vi "Aero_Tunnel_Monitor.vi"() -> ()   [LabVIEW 2012]
uses:
  ATE_Road_Data.ctl
  ATE_Machine_Status.ctl
  ATE_Road_Control.ctl
  ATE_Balance_Data.ctl
  ATE_Fan_Control.ctl
  ATE_Fan_Data.ctl
  Controls/Post_Process.ctl
  <vilib>/Platform/TimedLoop/XDataNode/timing_clust.ctl
  <vilib>/Platform/TimedLoop/XDataNode/nitl_modes.ctl
  <vilib>/Platform/TimedLoop/XDataNode/wakeup.ctl
  ADAM Client/Sub VIs/ADAM Controls/Update_scan_value.ctl
  Globals/Meas_global.vi
  <vilib>/Platform/TimedLoop/XDataNode/XDataNode.xnode
  <vilib>/Platform/TimedLoop/XDataNode/XDNodeRunTimeDep.lvlib
panel:
  out "Dem Tunnel Speed":dbl
  out "Paths":path[](array[path])
  out "error out":errorcluster
  out "Road Data REF":refnum<k21>="ni.var.psp://192.168.8.2/ATE_Shared_Variables/Road_Data"
  out "Road Control REF":refnum<k21>="ni.var.psp://192.168.8.2/ATE_Shared_Variables/Road_Control"
  out "Fan Data REF":refnum<k21>="ni.var.psp://192.168.8.2/ATE_Shared_Variables/Fan_Data"
  out "Fan Control REF":refnum<k21>="ni.var.psp://192.168.8.2/ATE_Shared_Variables/Fan_Control"
  out "Balance Data REF":refnum<k21>="ni.var.psp://192.168.8.2/ATE_Shared_Variables/Balance_Data"
  out "ATE_Machine Status REF":refnum<k21>="ni.var.psp://192.168.8.2/ATE_Shared_Variables/ATE_Machine_Status"
  in  "Stop Button":bool
  out "SMAD Temp":dbl=22.85
  out "First Loop? 3":bool
  out "First Loop? 2":bool
  out "First Loop?":bool=TRUE
  out "Fan Data":T1={"Fan Speed Dial (RPM)"=1.0, "Wind Speed Dial (m/s)"=0.0, "Wind Speed (m/s)"=0.0, "Fan Speed (RPM)"=1.0} {"Wind Speed Dial (m/s)" scale=0.0..45.0; "Fan Speed Dial (RPM)" scale=0.0..1000.0}
  out "Fan Control":T2={"Reset Pitot?"=FALSE, "Set Fan State"=FALSE, "Set Pressure"=1006.6041, "Set Fan Speed"=0.0, "Set Wind Speed Ratio"=1.0, "Tweak Change?"=FALSE, "Speed Change?"=FALSE}
  out "Balance_Data":T3={"%Lift"=28.01, "Lift"=185.018, "%Pitch"=22.34, "Pitch"=18.53, "%Drag"=2.21, "Drag"=4.327, "%Side"=-0.01, "Side"=-0.05, "%Yaw"=-2.47, "Yaw"=-0.307, "%Roll"=0.55, "Roll"=0.455} {"%Roll" scale=-100.0..100.0; "Roll" format="%5.1f Nm"; "%Yaw" scale=-100.0..100.0; "Yaw" format="%5.1f Nm"; "%Side" scale=-100.0..100.0; "Side" format="%5.1f N"; "%Drag" scale=-100.0..100.0; "Drag" format="%5.1f N"; "%Pitch" scale=-100.0..100.0; "Pitch" format="%5.1f Nm"; "%Lift" scale=-100.0..100.0; "Lift" format="%5.1f N"}
  in  "Road Control":T4 {"BL Suction Fan 2" scale=0.0..100.0; "BL Suction Fan 1" scale=0.0..100.0}
  out "ATE_Machine_Status":T5={"Loop Status"=FALSE, "Loop Frequency"=321.8613369862449, "Poor Loops"=0.0, "Pulse"=TRUE} {"Poor Loops" format="%0.2f %"; "Loop Frequency" format="%0.2f Hz"}
  out "Motor Enable":bool=TRUE
  out "Fan Watchdog":bool
  in  "Display Graph?":bool
  out "Belt Slip Warning":bool
  out "Road Enabled":bool
  out "Working Section Temperature":dbl=23.0
  out "Dem Road Speed":dbl
  in  "Balance Safety Limits":T6(array[cluster])=[{"Max +ve Range"=80, "Min -ve Range"=80, "Axis"="Lift"}, {"Max +ve Range"=80, "Min -ve Range"=80, "Axis"="Pitch"}, {"Max +ve Range"=120, "Min -ve Range"=120, "Axis"="Drag"}, {"Max +ve Range"=80, "Min -ve Range"=80, "Axis"="Side"}, {"Max +ve Range"=120, "Min -ve Range"=120, "Axis"="Yaw"}, {"Max +ve Range"=80, "Min -ve Range"=80, "Axis"="Roll"}]
  in  "Menu Ring":u16(ring) items=["Lift", "Pitch", "Drag", "Side", "Yaw", "Roll"]
  out "Waveform Chart":dbl(graph)
  out "OGI Client Loop Status":T5={"Loop Status"=FALSE, "Loop Frequency"=341.33991618739697, "Poor Loops"=1.2012012012012012, "Pulse"=FALSE} {"Poor Loops" format="%0.2f %"; "Loop Frequency" format="%0.2f Hz"}
  out "Road_Data":T7 {"Road Speed" scale=0.0..50.0; "Yaw Angle" scale=-5.0..5.0}
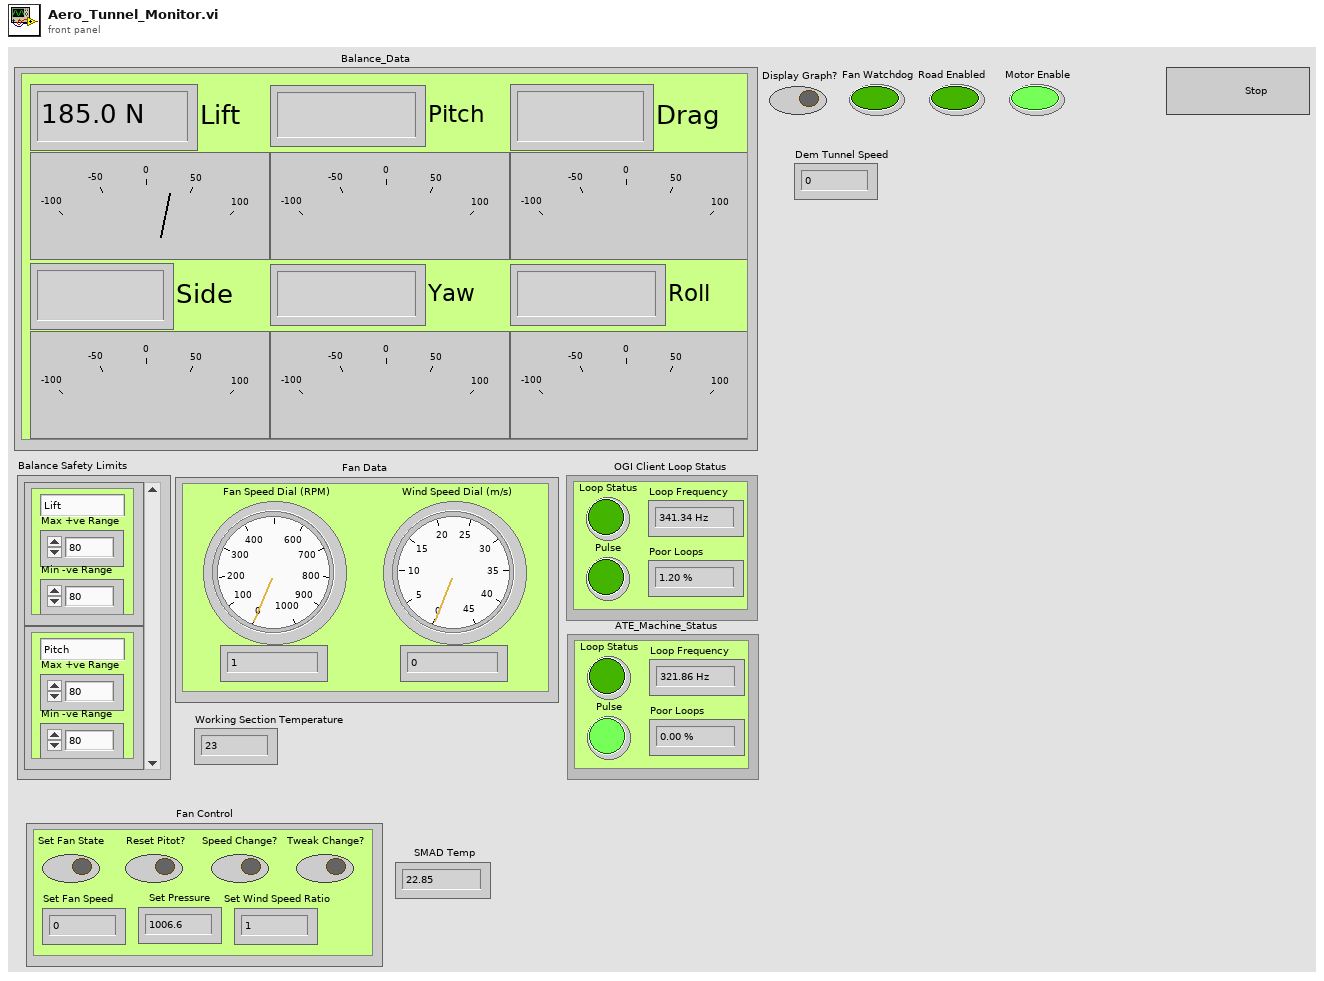
[diagram p1: front panel]
types:
  T1 = cluster{"Fan Speed Dial (RPM)":dbl, "Wind Speed Dial (m/s)":dbl, "Wind Speed (m/s)":dbl, "Fan Speed (RPM)":dbl}
  T2 = typedef "ATE_Fan_Control.ctl" = cluster{"Reset Pitot?":bool, "Set Fan State":bool, "Set Pressure":dbl, "Set Fan Speed":dbl, "Set Wind Speed Ratio":dbl, "Tweak Change?":bool, "Speed Change?":bool}
  T3 = typedef "ATE_Balance_Data.ctl" = cluster{"%Lift":dbl, "Lift":dbl, "%Pitch":dbl, "Pitch":dbl, "%Drag":dbl, "Drag":dbl, "%Side":dbl, "Side":dbl, "%Yaw":dbl, "Yaw":dbl, "%Roll":dbl, "Roll":dbl}
  T4 = typedef "ATE_Road_Control.ctl" = cluster{"Sync to Wind":bool, "Start Drive":bool, "Stop Drive":bool, "BL Suction Fan 1":i32, "BL Suction Fan 2":i32, "Set Yaw Angle":dbl, "Road Active?":bool}
  T5 = typedef "ATE_Machine_Status.ctl" = cluster{"Loop Status":bool, "Loop Frequency":dbl, "Poor Loops":dbl, "Pulse":bool}
  T6 = cluster{"Max +ve Range":i32, "Min -ve Range":i32, "Axis":string}[]
  T7 = typedef "ATE_Road_Data.ctl" = cluster{"Road Information":string, "Road Status":string, "Yaw Angle":dbl, "Road Speed":dbl}
  T8 = typedef "Post_Process.ctl" = enum16{"Take New Data", "Post Process Raw Data File"}
  T9 = typedef "Update_scan_value.ctl" = cluster{"Channel Name":string, "New Value":dbl}
  T10 = typedef "XDNodeRunTimeDep.lvlib/timing_clust.ctl" = cluster{"Expected End [f-1]":u64, "Actual End [f-1]":u64, "Finished Late? [f-1]":bool, "Expected End [i-1]":u64, "Actual End [i-1]":u64, "Finished Late? [i-1]":bool, "Expected Start [i]":u64, "Actual Start [i]":u64, "Expected Start [f]":u64, "Actual Start [f]":u64, "Source Name":string, "Structure Name":string, "Period":i64, "Deadline":i64, "Offset":i64, "Start":i64, "Priority":i32, "Timeout":i32, "Mode":T11, "Wakeup Reason":T12, "Error":errorcluster, "Source Type":string, "Secondary Source Type":string, "Global End Time":u64, "Global Start Time":u64, "Frame Duration":u64, "Iteration Duration":u64, "Assigned CPU":i32, "I/O Scan Engine Mode":u32}
  T11 = typedef "XDNodeRunTimeDep.lvlib/nitl_modes.ctl" = enum32{"No Change", "Process missed periods, maintain original phase", "Discard missed periods, maintain original phase", "Process missed periods, ignore original phase", "Discard missed periods, ignore original phase"}
  T12 = typedef "XDNodeRunTimeDep.lvlib/wakeup.ctl" = enum32{"Normal", "Aborted", "Asynchronous wakeup", "Timing source error", "Timed loop error", "Timeout"}
  T13 = typedef "ATE_Fan_Data.ctl" = cluster{"Fan Speed (RPM)":dbl, "Wind Speed (m/s)":dbl, "SMAD Data":string}
  T14 = typedef "LVDateTimeRec.ctl" = cluster{"fractional second":dbl, "second":i32, "minute":i32, "hour":i32, "day of month":i32, "month":i32, "year":i32, "day of week":i32, "day of year":i32, "DST":i32}
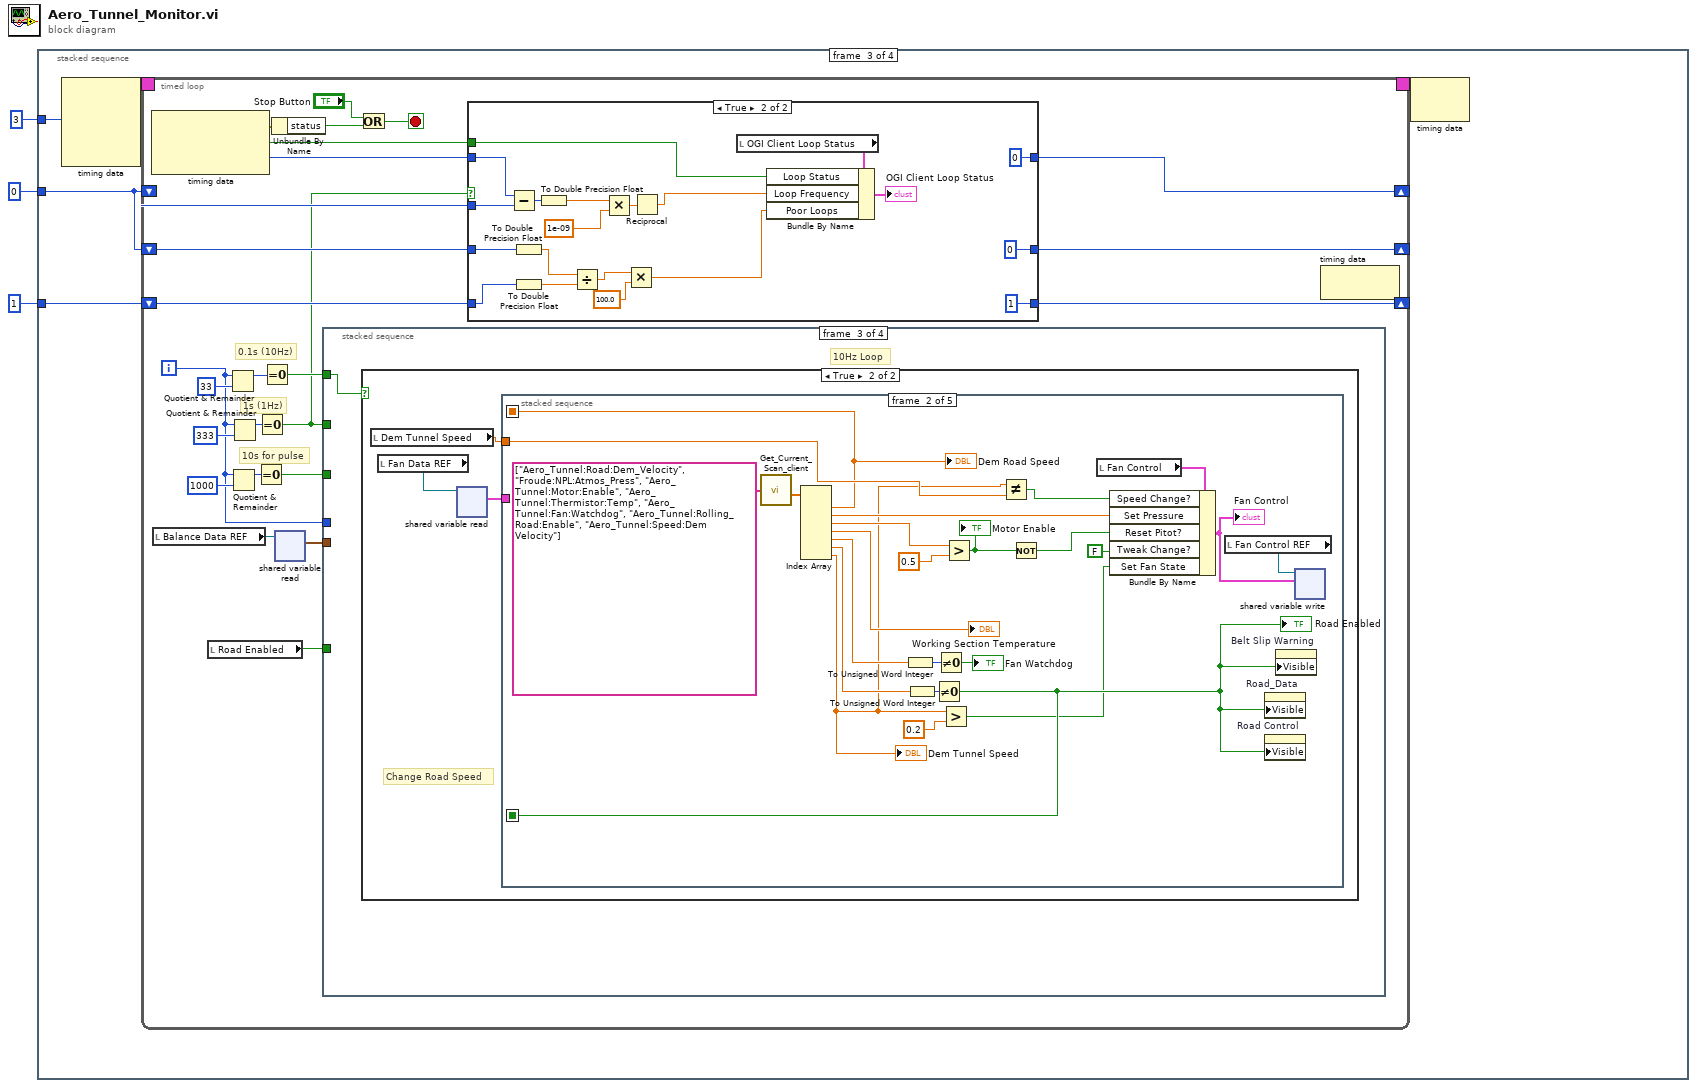
[diagram p0: block diagram]
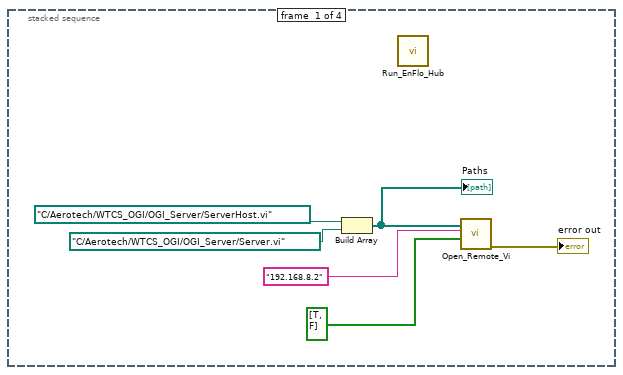
[diagram p2: hidden frame]
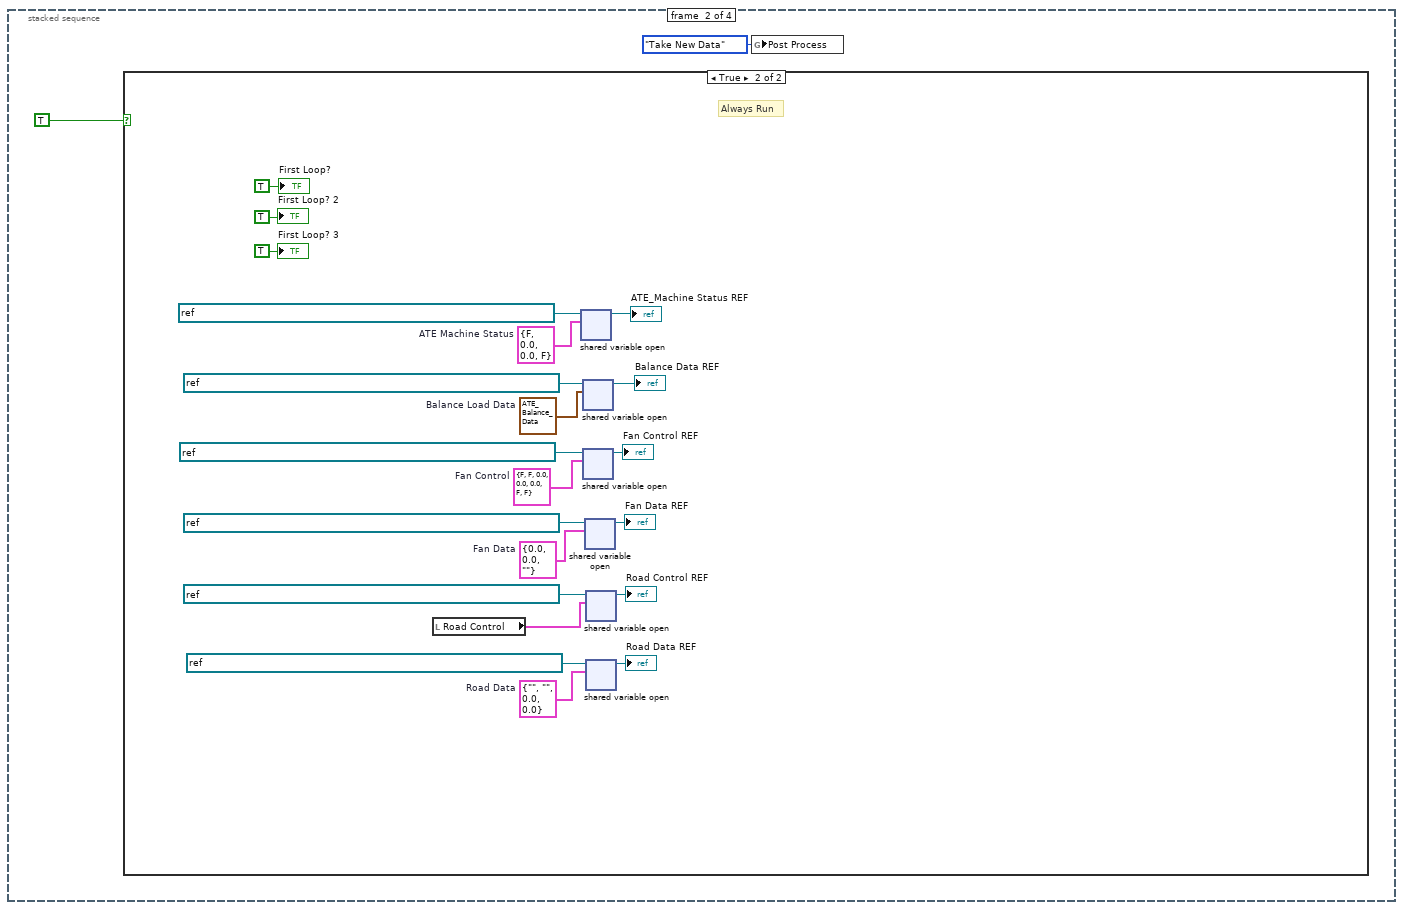
[diagram p3: hidden frame]
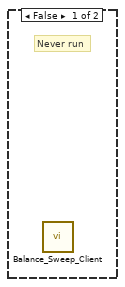
[diagram p4: hidden frame]
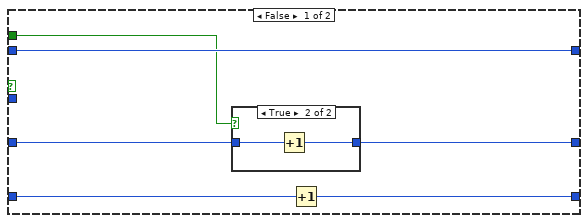
[diagram p5: hidden frame]
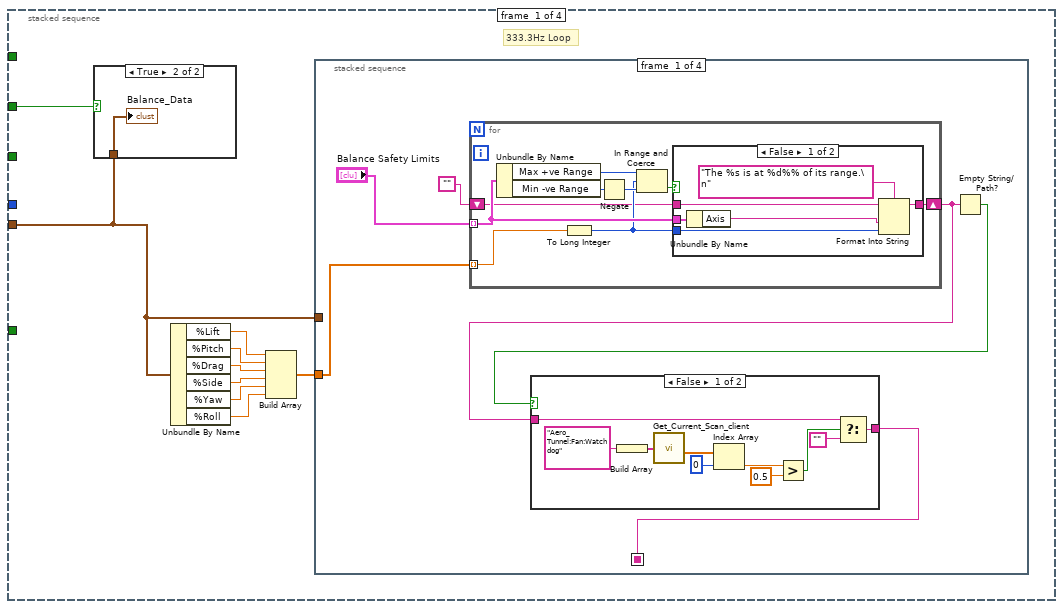
[diagram p7: hidden frame]
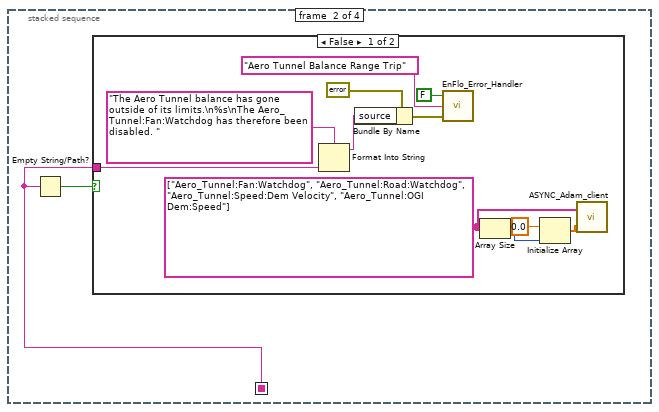
[diagram p11: hidden frame]
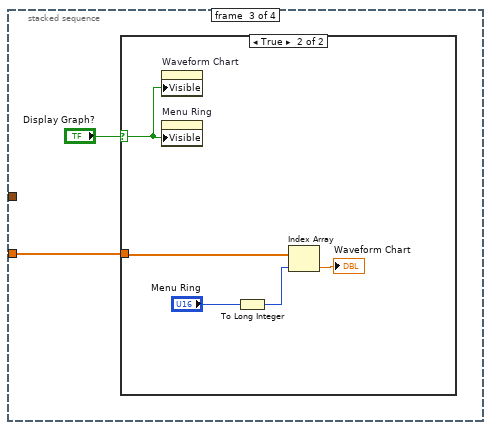
[diagram p13: hidden frame]
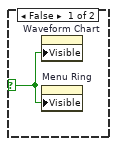
[diagram p14: hidden frame]
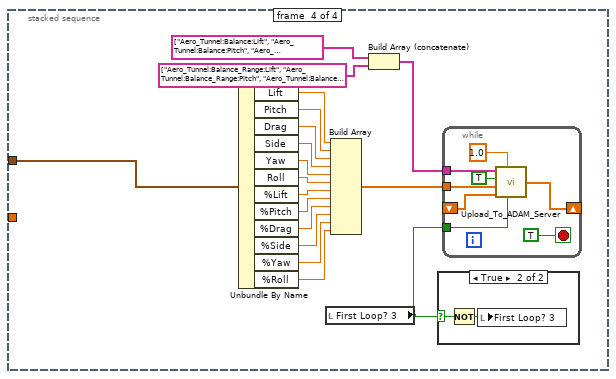
[diagram p15: hidden frame]
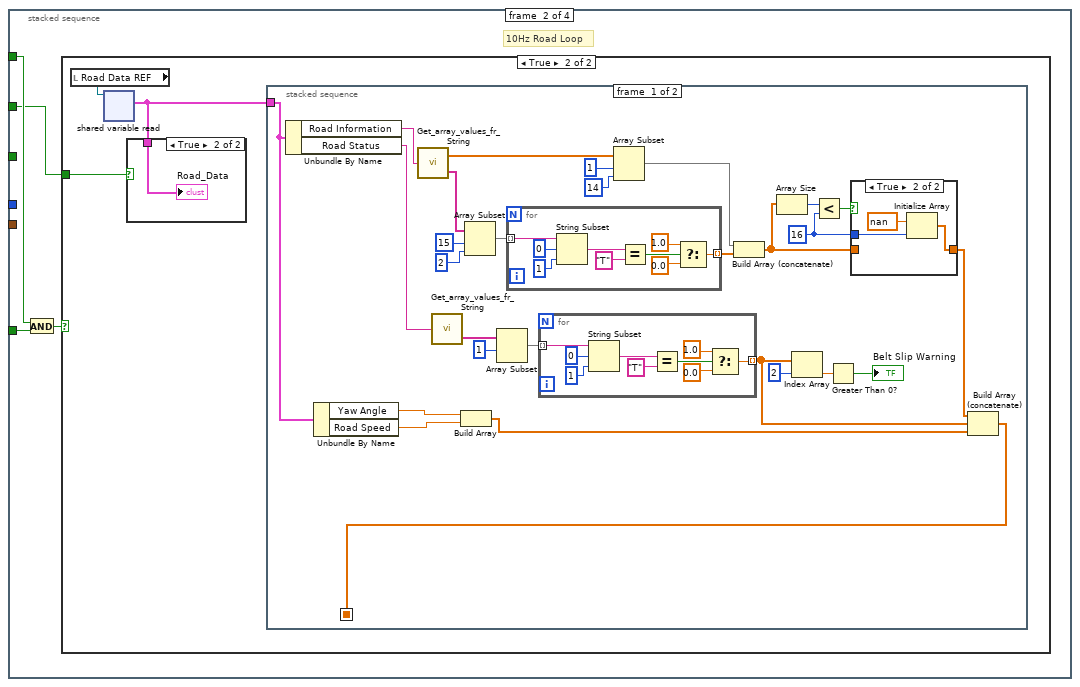
[diagram p17: hidden frame]
diagram:
  n1 = stacked-sequence {
    tunnel: i64 3 ("Period") -> [_ _ w35 _]
    tunnel: i64 0 ("Period") -> [_ _ w34 _]
    tunnel: i64 1 ("Period") -> [_ _ w33 _]
    frame #0 {
      n2 = Build Array(path "C:/Aerotech/WTCS_OGI/OGI_Server/ServerHost.vi" ("VI Path"), path "C:/Aerotech/WTCS_OGI/OGI_Server/Server.vi" ("VI Path")) -> (w6:path[])
      "Paths" <- w6
      n3 = call "Run_EnFlo_Hub.vi"() -> ()  [unwired: 8 in]
      n4 = call "Open_Remote_Vi.vi"("Run Minimised?"=bool[] [TRUE, FALSE], "Remote IP"="192.168.8.2", "Vi Path"=w6) -> ("error out"=→"error out":errorcluster)  [unwired: 8 in]
    }
    frame #1 {
      n5 = case shown="True" TRUE {
        frame False {
          # "Never run"
          n6 = call "Balance_Sweep_Client.vi"() -> ()  [unwired: 5 in, 1 out]
        }
        frame True {
          w17 = T7 {"Road Information"="", "Road Status"="", "Yaw Angle"=0.0, "Road Speed"=0.0}  # Road Data
          w28 = T5 {"Loop Status"=FALSE, "Loop Frequency"=0.0, "Poor Loops"=0.0, "Pulse"=FALSE}  # ATE Machine Status
          w20 = T13 {"Fan Speed (RPM)"=0.0, "Wind Speed (m/s)"=0.0, "SMAD Data"=""}  # Fan Data
          w22 = T2 {"Reset Pitot?"=FALSE, "Set Fan State"=FALSE, "Set Pressure"=0.0, "Set Fan Speed"=0.0, "Set Wind Speed Ratio"=0.0, "Tweak Change?"=FALSE, "Speed Change?"=FALSE}  # Fan Control
          w26 = T3 {"%Lift"=0.0, "Lift"=0.0, "%Pitch"=0.0, "Pitch"=0.0, "%Drag"=0.0, "Drag"=0.0, "%Side"=0.0, "Side"=0.0, "%Yaw"=0.0, "Yaw"=0.0, "%Roll"=0.0, "Roll"=0.0}  # Balance Load Data
          # "Always Run"
          n7 = local read "Road Control"() -> (w12:T4)
          n8 = shared-variable-open(refnum<k21> "ni.var.psp://192.168.8.2/ATE_Shared_Variables/ATE_Machine_Status" ("shared variable refnum in"), w28) -> (→"ATE_Machine Status REF":refnum<k21>)  [unwired: 2 in, 1 out]
          n9 = shared-variable-open(refnum<k21> "ni.var.psp://192.168.8.2/ATE_Shared_Variables/Balance_Data" ("shared variable refnum in"), w26) -> (→"Balance Data REF":refnum<k21>)  [unwired: 2 in, 1 out]
          n10 = shared-variable-open(refnum<k21> "ni.var.psp://192.168.8.2/ATE_Shared_Variables/Fan_Control" ("shared variable refnum in"), w22) -> (→"Fan Control REF":refnum<k21>)  [unwired: 2 in, 1 out]
          n11 = shared-variable-open(refnum<k21> "ni.var.psp://192.168.8.2/ATE_Shared_Variables/Fan_Data" ("shared variable refnum in"), w20) -> (→"Fan Data REF":refnum<k21>)  [unwired: 2 in, 1 out]
          n12 = shared-variable-open(refnum<k21> "ni.var.psp://192.168.8.2/ATE_Shared_Variables/Road_Control" ("shared variable refnum in"), w12) -> (→"Road Control REF":refnum<k21>)  [unwired: 2 in, 1 out]
          n13 = shared-variable-open(refnum<k21> "ni.var.psp://192.168.8.2/ATE_Shared_Variables/Road_Data" ("shared variable refnum in"), w17) -> (→"Road Data REF":refnum<k21>)  [unwired: 2 in, 1 out]
          "First Loop?" <- TRUE
          "First Loop? 2" <- TRUE
          "First Loop? 3" <- TRUE
        }
      }
      n14 = global write "Meas_global.vi" "Post Process"(Post_Process."Take New Data" ("Post Process")) -> ()
    }
    frame #2 {
      n15 = node-c288(w35) -> (w37:T10)  [unwired: 3 in]
      n16 = timed-loop {
        timing: w37 -> [_]
        timing-out: [_] -> w36
        shift-right: [w44] -> _
        shift-left: w34 -> [w51]
        shift-right: [w46] -> _
        shift-left: w34 -> [w58]
        shift-right: [w49] -> _
        shift-left: w33 -> [w48]
        i -> [w38]
        stop <- w41 stop-if-true
        # "10s for pulse"
        # "1s (1Hz)"
        # "0.1s (10Hz)"
        n17 = node-c288() -> (w62:errorcluster, w47:bool, w59:i64)  [unwired: 1 in]
        n18 = local read "Balance Data REF"() -> (w40:refnum<k21>)
        n19 = local read "Road Enabled"() -> (w55:bool)
        n20 = Quotient & Remainder(x=w38, y=33) -> (x-y*floor(x/y)=w60:i32)  [unwired: 1 out]
        n21 = Quotient & Remainder(x=w38, y=1000) -> (x-y*floor(x/y)=w56:i32)  [unwired: 1 out]
        n22 = Quotient & Remainder(x=w38, y=333) -> (x-y*floor(x/y)=w61:i32)  [unwired: 1 out]
        n23 = Equal To 0?(x=w56) -> (x = 0?=w50:bool)
        n24 = Equal To 0?(x=w61) -> (x = 0?=w45:bool)
        n25 = Equal To 0?(x=w60) -> (x = 0?=w57:bool)
        n26 = Unbundle By Name(w62) -> ("status"=w43:bool)
        n27 = shared-variable-read(w40) -> (w39:T3)  [unwired: 1 in, 3 out]
        n28 = stacked-sequence {
          tunnel: w57 -> [_ w185 w259 _]
          tunnel: w45 -> [w93 w184 _ _]
          tunnel: w55 -> [_ w186 _ _]
          tunnel: w50 -> [_ _ _ w367]
          tunnel: w39 -> [w92 _ _ _]
          tunnel: w38 -> [_ _ _ w366]
          frame #0 {
            # "333.3Hz Loop"
            n29 = case shown="True" w93 {
              tunnel: w92 -> [_ w101]
              frame False {
              }
              frame True {
                "Balance_Data" <- w101
              }
            }
            n30 = Unbundle By Name(w92) -> ("%Lift"=w99:dbl, "%Pitch"=w98:dbl, "%Drag"=w97:dbl, "%Side"=w96:dbl, "%Yaw"=w95:dbl, "%Roll"=w94:dbl)
            n31 = Build Array(w99, w98, w97, w96, w95, w94) -> (w100:dbl[])
            n32 = stacked-sequence {
              seq-local: [w102 _ _ _] -> [_ w135 _ _]
              tunnel: w100 -> [w106 _ w148 _]
              tunnel: w92 -> [_ _ _ w159]
              frame #0 {
                n33 = for {
                  tunnel: "Balance Safety Limits" -> [w122] mode=indexing
                  tunnel: w106 -> [w125] mode=indexing
                  shift-right: [w119] -> w104
                  shift-left: "" -> [w120]
                  n34 = Unbundle By Name(w122) -> ("Max +ve Range"=w127:i32, "Min -ve Range"=w126:i32)
                  n35 = To Long Integer(number=w125) -> (32bit integer=w121:i32)
                  n36 = Negate(x=w126) -> (-x=w124:i32)
                  n37 = In Range and Coerce(upper limit=w127, x=w121, lower limit=w124) -> (In Range?=w123:bool)  [unwired: 1 out]
                  n38 = case shown="False" w123 {
                    tunnel: w122 -> [w133 _]
                    tunnel: w121 -> [w131 _]
                    tunnel: w120 -> [w129 w134]
                    tunnel: [w128 w134] -> w119
                    frame False {
                      n39 = Unbundle By Name(w133) -> ("Axis"=w132:string)
                      n40 = Format Into String(format string="The %s is at %d%% of its range.\n", initial string=w129, w132, w131) -> (resulting string=w128:string)  [unwired: 1 in, 1 out]
                    }
                    frame True {
                    }
                  }
                }
                n41 = Empty String/Path?(string/path=w104) -> (empty?=w105:bool)
                n42 = case shown="False" w105 {
                  tunnel: w104 -> [w110 w118]
                  tunnel: [w108 w118] -> w102
                  frame False {
                    n43 = Build Array("Aero_Tunnel:Fan:Watchdog") -> (w117:string[])
                    n44 = call "Get_Current_Scan_client.vi"("ADAM Ch Names"=w117) -> ("Numerical Values"=w115:dbl[])  [unwired: 1 in, 2 out]
                    n45 = Index Array(array=w115, index=0) -> (element=w113:dbl)
                    n46 = Greater?(x=w113, y=0.5) -> (0:w111:bool)
                    n47 = Select(t=w110, s=w111, f="") -> (s? t:f=w108:string)
                  }
                  frame True {
                  }
                }
              }
              frame #1 {
                n48 = Empty String/Path?(string/path=w135) -> (empty?=w136:bool)
                n49 = case shown="False" w136 {
                  tunnel: w135 -> [w141 _]
                  frame False {
                    w140 = string[] ["Aero_Tunnel:Fan:Watchdog", "Aero_Tunnel:Road:Watchdog", "Aero_Tunnel:Speed:Dem Velocity", "Aero_Tunnel:OGI Dem:Speed"] ("Channel Names")
                    n50 = Format Into String(format string="The Aero Tunnel balance has gone outside of its limits.\n%s\nThe Aero_Tunnel:Fan:Watchdog has therefore been disabled. ", w141) -> (resulting string=w142:string)  [unwired: 2 in, 1 out]
                    n51 = Bundle By Name(cluster=errorcluster {"status"=TRUE, "code"=0, "source"=""} ("error in (no error)"), "source"=w142) -> (w144:errorcluster)
                    n52 = call "EnFlo_Error_Handler.vi"("error in (no error)"=w144, "Error Type"="Aero Tunnel Balance Range Trip", "Dialog Box (T)"=FALSE) -> ()  [unwired: 3 out]
                    n53 = Array Size(array=w140) -> (size(s)=w139:i32)
                    n54 = Initialize Array(0.0, w139) -> (w137:dbl[])
                    n55 = call "ASYNC_Adam_client.vi"("Values"=w137, "Channel Names"=w140) -> ()  [unwired: 2 out]
                  }
                  frame True {
                  }
                }
              }
              frame #2 {
                n56 = case shown="True" "Display Graph?" {
                  selector: "Display Graph?" -> [w150 w153]
                  tunnel: w148 -> [_ w151]
                  frame False {
                    n57 = property on="Waveform Chart" class="WFChart (strict)"("Visible"=w150) -> ()  [unwired: 2 in, 2 out]
                    n58 = property on="Menu Ring" class="Ring (strict)"("Visible"=w150) -> ()  [unwired: 2 in, 2 out]
                  }
                  frame True {
                    n59 = property on="Waveform Chart" class="WFChart (strict)"("Visible"=w153) -> ()  [unwired: 2 in, 2 out]
                    n60 = property on="Menu Ring" class="Ring (strict)"("Visible"=w153) -> ()  [unwired: 2 in, 2 out]
                    n61 = To Long Integer(number="Menu Ring") -> (32bit integer=w152:i32)
                    n62 = Index Array(array=w151, index=w152) -> (element=→"Waveform Chart":dbl)
                  }
                }
              }
              frame #3 {
                n63 = Unbundle By Name(w159) -> ("Lift"=w173:dbl, "Pitch"=w172:dbl, "Drag"=w171:dbl, "Side"=w170:dbl, "Yaw"=w169:dbl, "Roll"=w168:dbl, "%Lift"=w167:dbl, "%Pitch"=w166:dbl, "%Drag"=w165:dbl, "%Side"=w164:dbl, "%Yaw"=w163:dbl, "%Roll"=w162:dbl)
                n64 = local read "First Loop? 3"() -> (w156:bool)
                n65 = Build Array(w173, w172, w171, w170, w169, w168, w167, w166, w165, w164, w163, w162) -> (w157:dbl[])
                n66 = Build Array (concatenate)(string[] ["Aero_Tunnel:Balance:Lift", "Aero_Tunnel:Balance:Pitch", "Aero_Tunnel:Balance:Drag", "Aero_Tunnel:Balance:Side-Force", "Aero_Tunnel:Balance:Yaw", "Aero_Tunnel:Balance:Roll"] ("Channel Names"), string[] ["Aero_Tunnel:Balance_Range:Lift", "Aero_Tunnel:Balance_Range:Pitch", "Aero_Tunnel:Balance_Range:Drag", "Aero_Tunnel:Balance_Range:Side-Force", "Aero_Tunnel:Balance_Range:Yaw", "Aero_Tunnel:Balance_Range:Roll"] ("Channel Names")) -> (w158:string[])
                n67 = case shown="True" w156 {
                  selector: w156 -> [_ w175]
                  frame False {
                  }
                  frame True {
                    n68 = Not(x=w175) -> (.not. x?=w174:bool)
                    n69 = local write "First Loop? 3"(w174) -> ()
                  }
                }
                n70 = while {
                  tunnel: w158 -> [w183]
                  tunnel: w157 -> [w181]
                  shift-right: [w179] -> _
                  shift-left: _ -> [w178]
                  tunnel: w156 -> [w177]
                  stop <- TRUE stop-if-true
                  n71 = call "Upload_To_ADAM_Server.vi"("First Loop"=w177, "Averaging Period (s)"=1.0, "Shift In"=w178, "Channel Values"=w181, "Give Variance"=TRUE, "Channel Names"=w183) -> ("Shift Out"=w179:dbl[])
                }
              }
            }
          }
          frame #1 {
            # "10Hz Road Loop"
            n72 = And(x=w185, y=w186) -> (x .and. y?=w187:bool)
            n73 = case shown="True" w187 {
              tunnel: w184 -> [_ w190]
              frame False {
                # "Do Nothing"
              }
              frame True {
                n74 = local read "Road Data REF"() -> (w189:refnum<k21>)
                n75 = shared-variable-read(w189) -> (w188:T7)  [unwired: 1 in, 3 out]
                n76 = case shown="True" w190 {
                  tunnel: w188 -> [_ w191]
                  frame False {
                  }
                  frame True {
                    "Road_Data" <- w191
                  }
                }
                n77 = stacked-sequence {
                  seq-local: [w196 _] -> [_ w245]
                  tunnel: w188 -> [w195 _]
                  frame #0 {
                    w217 = 16 ("y")
                    n78 = Unbundle By Name(w195) -> ("Road Information"=w206:string, "Road Status"=w200:string)
                    n79 = Unbundle By Name(w195) -> ("Yaw Angle"=w194:dbl, "Road Speed"=w193:dbl)
                    n80 = call "Get_array_values_fr_String.vi"("String Value"=w206) -> ("Numeric Array"=w218:dbl[], "String array"=w214:string[])
                    n81 = call "Get_array_values_fr_String.vi"("String Value"=w200) -> ("String array"=w203:string[])  [unwired: 1 out]
                    n82 = Build Array(w194, w193) -> (w192:dbl[])
                    n83 = Array Subset(array=w214, index=15, length=2) -> (w211:string[])
                    n84 = Array Subset(array=w203, index=1) -> (w205:string[])  [unwired: 1 in]
                    n85 = for {
                      tunnel: w211 -> [w239] mode=indexing
                      tunnel: [w233] -> w212 mode=indexing
                      n86 = String Subset(string=w239, offset (0)=0, length (rest)=1 ("length (rest)")) -> (substring=w238:string)
                      n87 = Equal?(x=w238, y="T") -> (x = y?=w236:bool)
                      n88 = Select(t=1.0, s=w236, f=0.0) -> (s? t:f=w233:dbl)
                    }
                    n89 = for {
                      tunnel: [w221] -> w197 mode=indexing
                      tunnel: w205 -> [w220] mode=indexing
                      n90 = String Subset(string=w220, offset (0)=0, length (rest)=1 ("length (rest)")) -> (substring=w226:string)
                      n91 = Equal?(x=w226, y="T") -> (x = y?=w224:bool)
                      n92 = Select(t=1.0, s=w224, f=0.0) -> (s? t:f=w221:dbl)
                    }
                    n93 = Array Subset(array=w218, index=1, length=14) -> (w213:dbl[])
                    n94 = Build Array (concatenate)(w213, w212) -> (w219:dbl[])
                    n95 = Array Size(array=w219) -> (size(s)=w215:i32)
                    n96 = Index Array(array=w197, index=2) -> (element=w202:dbl)
                    n97 = Less?(x=w215, y=w217) -> (x < y?=w216:bool)
                    n98 = Greater Than 0?(x=w202) -> (x > 0?=→"Belt Slip Warning":bool)
                    n99 = case shown="True" w216 {
                      tunnel: [w229 w232] -> w198
                      tunnel: w219 -> [w229 _]
                      tunnel: w217 -> [_ w230]
                      frame False {
                      }
                      frame True {
                        n100 = Initialize Array(nan, w230) -> (w232:dbl[])
                      }
                    }
                    n101 = Build Array (concatenate)(w198, w197, w192) -> (w196:dbl[])
                  }
                  frame #1 {
                    n102 = Build Array (concatenate)(string[] ["Aero_Tunnel:Road_Belt:Travel_km", "Aero_Tunnel:Road_Platen_Temp:Front_Left", "Aero_Tunnel:Road_Platen_Temp:Front_Right", "Aero_Tunnel:Road_Platen_Temp:Rear_Left", "Aero_Tunnel:Road_Platen_Temp:Rear_Right", "Aero_Tunnel:Road_Water:Outlet _Temp", "Aero_Tunnel:Road_Water:Inlet _Temp", "Aero_Tunnel:Road_Suction:Front", "Aero_Tunnel:Road_Suction:Middle", "Aero_Tunnel:Road_Suction:Rear", "Aero_Tunnel:Road_BL_Suction:Primary", "Aero_Tunnel:Road_BL_Suction:Secondary", "Aero_Tunnel:Road_LoadCell:Left", "Aero_Tunnel:Road_LoadCell:Right", "Aero_Tunnel:Road_Water_High:Temp_Alarm", "Aero_Tunnel:Road_Platen_High:Temp_Alarm"] ("Channel Names"), string[] ["Aero_Tunnel:Road_E-Stop:Active", "Aero_Tunnel:Road_Main_Drives:Started", "Aero_Tunnel:Road_Belt_Slip:Warning", "Aero_Tunnel:Road_Belt_Absent:or_Broken", "Aero_Tunnel:Road_Suction:Established", "Aero_Tunnel:Road_Load_Error:Left", "Aero_Tunnel:Road_Load_Error:Right", "Aero_Tunnel:Road_Water_Alarm:Active", "Aero_Tunnel:Road_Platen_Alarm:Active"] ("Channel Names"), string[] ["Aero_Tunnel:Road_Yaw:Angle_Deg", "Aero_Tunnel:Road_Speed:m/s"] ("Channel Names")) -> (w246:string[])
                    n103 = local read "First Loop?"() -> (w244:bool)
                    n104 = while {
                      tunnel: w246 -> [w258]
                      tunnel: w245 -> [w256]
                      shift-right: [w254] -> _
                      shift-left: _ -> [w253]
                      tunnel: w244 -> [w252]
                      stop <- TRUE stop-if-true
                      n105 = call "Upload_To_ADAM_Server.vi"("First Loop"=w252, "Averaging Period (s)"=1.0, "Shift In"=w253, "Channel Values"=w256, "Channel Names"=w258) -> ("Shift Out"=w254:dbl[])  [unwired: 1 in]
                    }
                    n106 = case shown="True" w244 {
                      selector: w244 -> [_ w251]
                      frame False {
                      }
                      frame True {
                        n107 = Not(x=w251) -> (.not. x?=w250:bool)
                        n108 = local write "First Loop?"(w250) -> ()
                      }
                    }
                    n109 = local read "Road Control REF"() -> (w243:refnum<k21>)
                    n110 = shared-variable-write(w243, "Road Control") -> ()  [unwired: 1 in, 2 out]
                  }
                }
              }
            }
          }
          frame #2 {
            # "10Hz Loop"
            n111 = case shown="True" w259 {
              frame False {
                # "Do Nothing"
              }
              frame True {
                # "Change Road Speed"
                n112 = local read "Dem Tunnel Speed"() -> (w260:dbl)
                n113 = local read "Fan Data REF"() -> (w262:refnum<k21>)
                n114 = shared-variable-read(w262) -> (w261:T13)  [unwired: 1 in, 3 out]
                n115 = stacked-sequence {
                  seq-local: [_ w307 _ _ _] -> [_ _ w333 _ _]
                  seq-local: [_ w304 _ _ _] -> [_ _ w328 _ _]
                  tunnel: w261 -> [w285 _ _ _ _]
                  tunnel: w260 -> [_ w306 _ _ _]
                  frame #0 {
                    w271 = 17 ("y")
                    n116 = Unbundle By Name(w285) -> ("Wind Speed (m/s)"=w267:dbl, "Fan Speed (RPM)"=w268:dbl, "SMAD Data"=w269:string)
                    n117 = call "Get_array_values_fr_String.vi"("String Value"=w269) -> ("Numeric Array"=w272:dbl[], "String array"=w275:string[])
                    n118 = Array Size(array=w275) -> (size(s)=w276:i32)
                    n119 = Less?(x=w276, y=w271) -> (x < y?=w274:bool)
                    n120 = case shown="True" w274 {
                      tunnel: [w290 w293] -> w273
                      tunnel: w272 -> [w290 _]
                      tunnel: w271 -> [_ w291]
                      frame False {
                      }
                      frame True {
                        n121 = Initialize Array(nan, w291) -> (w293:dbl[])
                      }
                    }
                    n122 = Bundle By Name(cluster=T1 {"Fan Speed Dial (RPM)"=143.0, "Wind Speed Dial (m/s)"=4.76, "Wind Speed (m/s)"=0.0, "Fan Speed (RPM)"=0.0} ("Fan Data"), "Wind Speed Dial (m/s)"=w267, "Fan Speed Dial (RPM)"=w268, "Wind Speed (m/s)"=w267, "Fan Speed (RPM)"=w268) -> (→"Fan Data":T1)
                    n123 = Index Array(array=w273, index=16) -> (element=w263:dbl)
                    "SMAD Temp" <- w263
                    n124 = Index Array(array=w273, index=1) -> (element=w282:dbl)
                    n125 = Index Array(array=w273, index=11) -> (element=w280:dbl)
                    n126 = Less?(x=w280, y=100.0) -> (x < y?=w278:bool)
                    n127 = Boolean To (0,1)(Boolean=w278) -> (0, 1=w277:i16)
                    n128 = Build Array(w263, w282, w277) -> (w270:dbl[])
                    n129 = local read "First Loop? 2"() -> (w266:bool)
                    n130 = Build Array (concatenate)(w267, w268, w270) -> (w286:dbl[])
                    n131 = case shown="True" w266 {
                      selector: w266 -> [_ w289]
                      frame False {
                      }
                      frame True {
                        n132 = Not(x=w289) -> (.not. x?=w288:bool)
                        n133 = local write "First Loop? 2"(w288) -> ()
                      }
                    }
                    n134 = while {
                      tunnel: string[] ["Aero_Tunnel:Speed:Meas Velocity", "Aero_Tunnel:Fan:RPM", "Aero_Tunnel:SmAD:Temp", "Aero_Tunnel:Pitot tube:Voltage", "Aero_Tunnel:Drive:Ready"] ("Channel Names") -> [w300]
                      tunnel: w286 -> [w298]
                      shift-right: [w297] -> _
                      shift-left: _ -> [w296]
                      tunnel: w266 -> [w294]
                      stop <- TRUE stop-if-true
                      n135 = call "Upload_To_ADAM_Server.vi"("First Loop"=w294, "Averaging Period (s)"=1.0, "Shift In"=w296, "Channel Values"=w298, "Channel Names"=w300) -> ("Shift Out"=w297:dbl[])  [unwired: 1 in]
                    }
                  }
                  frame #1 {
                    n136 = call "Get_Current_Scan_client.vi"("ADAM Ch Names"=string[] ["Aero_Tunnel:Road:Dem_Velocity", "Froude:NPL:Atmos_Press", "Aero_Tunnel:Motor:Enable", "Aero_Tunnel:Thermistor:Temp", "Aero_Tunnel:Fan:Watchdog", "Aero_Tunnel:Rolling_Road:Enable", "Aero_Tunnel:Speed:Dem Velocity"] ("appended array")) -> ("Numerical Values"=w323:dbl[])  [unwired: 1 in, 2 out]
                    n137 = Index Array(array=w323) -> (element #1=w304:dbl, element #2=w317:dbl, element #3=w318:dbl, element #4=→"Working Section Temperature":dbl, element #5=w309:dbl, element #6=w308:dbl, element #7=w302:dbl)  [unwired: 7 in]
                    "Dem Road Speed" <- w304
                    "Dem Tunnel Speed" <- w302
                    n138 = To Unsigned Word Integer(number=w309) -> (unsigned 16bit integer=w321:u16)
                    n139 = To Unsigned Word Integer(number=w308) -> (unsigned 16bit integer=w322:u16)
                    n140 = Not Equal To 0?(x=w322) -> (x != 0?=w307:bool)
                    "Road Enabled" <- w307
                    n141 = Not Equal To 0?(x=w321) -> (x != 0?=→"Fan Watchdog":bool)
                    n142 = Greater?(x=w302, y=0.2) -> (0:w303:bool)
                    n143 = Greater?(x=w318, y=0.5) -> (0:w315:bool)
                    "Motor Enable" <- w315
                    n144 = Not Equal?(x=w302, y=w306) -> (x != y?=w305:bool)
                    n145 = Not(x=w315) -> (.not. x?=w314:bool)
                    n146 = local read "Fan Control"() -> (w301:T2)
                    n147 = Bundle By Name(cluster=w301, "Speed Change?"=w305, "Set Pressure"=w317, "Reset Pitot?"=w314, "Tweak Change?"=FALSE, "Set Fan State"=w303) -> (w312:T2)
                    "Fan Control" <- w312
                    n148 = local read "Fan Control REF"() -> (w313:refnum<k21>)
                    n149 = property on="Road_Data" class="Clust (strict)"("Visible"=w307) -> ()  [unwired: 2 in, 2 out]
                    n150 = property on="Road Control" class="Clust (strict)"("Visible"=w307) -> ()  [unwired: 2 in, 2 out]
                    n151 = property on="Belt Slip Warning" class="Bool (strict)"("Visible"=w307) -> ()  [unwired: 2 in, 2 out]
                    n152 = shared-variable-write(w313, w312) -> ()  [unwired: 1 in, 2 out]
                  }
                  frame #2 {
                    n153 = Greater?(x=w328, y=0.3) -> (0:w326:bool)
                    n154 = Not(x=w326) -> (.not. x?=w325:bool)
                    n155 = local read "Road Control"() -> (w330:T4)
                    n156 = Bundle By Name(cluster=w330, "Road Active?"=w333, "Sync to Wind"=TRUE, "Start Drive"=w326, "Stop Drive"=w325) -> (w332:T4)
                    n157 = local read "Road Control REF"() -> (w331:refnum<k21>)
                    n158 = shared-variable-write(w331, w332) -> ()  [unwired: 1 in, 2 out]
                  }
                  frame #3 {
                    n159 = local read "Dem Tunnel Speed"() -> (w339:dbl)
                    n160 = call "Polynomial_convert.vi"("Calib constants"=dbl[] [1.1471940648, -0.0162969407, 0.0008616246, -2.02143e-05, 1.764e-07], "Voltage"=w339) -> ("Eng Values"=w344:dbl)  [unwired: 4 in]
                    n161 = Equal To 0?(x=w339) -> (x = 0?=w338:bool)
                    n162 = In Range and Coerce(upper limit=1.12, x=w344, lower limit=0.88) -> (coerced(x)=w337:dbl)  [unwired: 1 out]
                    n163 = local read "Dem Road Speed"() -> (w334:dbl)
                    n164 = Select(t=0.88, s=w338, f=w337) -> (s? t:f=w336:dbl)
                    n165 = local read "Fan Control"() -> (w342:T2)
                    n166 = Bundle By Name(cluster=w342, "Set Wind Speed Ratio"=w336, "Set Fan Speed"=w334) -> (w341:T2)
                    n167 = local read "Fan Control REF"() -> (w340:refnum<k21>)
                    n168 = shared-variable-write(w340, w341) -> ()  [unwired: 1 in, 2 out]
                  }
                  frame #4 {
                    n169 = while {
                      shift-right: [w348] -> _
                      shift-left: _ -> [w349]
                      stop <- TRUE stop-if-true
                      n170 = local read "Working Section Temperature"() -> (w347:dbl)
                      n171 = Greater?(x=w347, y=35.0) -> (0:w348:bool)
                      n172 = Compound Arithmetic op=AND(invert w349, w348) -> (w354:bool)
                      n173 = Number To Fractional String(number=w347, precision (6)=i16 2) -> (F-format string=w351:string)  [unwired: 2 in]
                      n174 = case shown="True" w354 {
                        tunnel: w351 -> [_ w359]
                        frame False {
                        }
                        frame True {
                          w358 = string[] ["Aero_Tunnel:Fan:Watchdog", "Aero_Tunnel:Road:Watchdog", "Aero_Tunnel:Speed:Dem Velocity", "Aero_Tunnel:OGI Dem:Speed"] ("Channel Names")
                          n175 = Format Into String(format string="The Aero Tunnel temperature has gone above it's limits and is:\n%s\nThe Aero_Tunnel:Fan:Watchdog has therefore been disabled. ", w359) -> (resulting string=w360:string)  [unwired: 2 in, 1 out]
                          n176 = Bundle By Name(cluster=errorcluster {"status"=TRUE, "code"=0, "source"=""} ("error in (no error)"), "source"=w360) -> (w362:errorcluster)
                          n177 = Array Size(array=w358) -> (size(s)=w357:i32)
                          n178 = call "EnFlo_Error_Handler.vi"("error in (no error)"=w362, "Error Type"="Aero Tunnel Temperature Trip", "Dialog Box (T)"=FALSE) -> ()  [unwired: 3 out]
                          n179 = Initialize Array(0.0, w357) -> (w355:dbl[])
                          n180 = call "ASYNC_Adam_client.vi"("Values"=w355, "Channel Names"=w358) -> ()  [unwired: 2 out]
                        }
                      }
                    }
                  }
                }
              }
            }
          }
          frame #3 {
            # "10s Loop For Pulse"
            n181 = case shown="True" w367 {
              tunnel: w366 -> [_ w368]
              frame False {
                # "Do Nothing"
              }
              frame True {
                n182 = while {
                  shift-right: [w373] -> _
                  shift-left: "Start" -> [w374]
                  shift-right: [w372] -> _
                  shift-left: _ -> [w371]
                  tunnel: w368 -> [w370]
                  stop <- w375 continue-if-true
                  n183 = case shown="\"Close Server\"" w374 {
                    tunnel: [FALSE TRUE TRUE TRUE TRUE FALSE] -> w375
                    tunnel: ["" "Check Pulse" "Check Pulse" w415 "ReOpen" ""] -> w373
                    tunnel: [w376 w382 0 ("code") w407 w443 w452] -> w372
                    tunnel: w371 -> [w376 w383 _ w404 w443 w452]
                    tunnel: w370 -> [_ w386 _ _ _ _]
                    frame "No Match", Default {
                    }
                    frame "Start" {
                      n184 = Greater?(x=w386, y=1500) -> (0:w381:bool)
                      n185 = while {
                        shift-right: [w390] -> _
                        shift-left: _ -> [w389]
                        stop <- TRUE stop-if-true
                        n186 = Seconds To Date/Time() -> (date time rec=w391:T14)  [unwired: 2 in]
                        n187 = Unbundle By Name(w391) -> ("day of year"=w390:i32)
                        n188 = Not Equal?(x=w390, y=w389) -> (x != y?=w388:bool)
                        n189 = case shown="True" w388 {
                          frame False {
                          }
                          frame True {
                            n190 = Get Date/Time In Seconds() -> (seconds since 1Jan1904=w393:timestamp)
                            n191 = To Double Precision Float(number=w393) -> (double precision float=w392:dbl)
                            n192 = global write "Meas_global.vi" "Start Time of experiment"(w392) -> ()
                          }
                        }
                      }
                      n193 = Select(t=w383, s=w381, f=0) -> (s? t:f=w382:i32)
                    }
                    frame "ReOpen" {
                      n194 = local read "Paths"() -> (w400:path[])
                      n195 = call "Open_Remote_Vi.vi"("Run Minimised?"=bool[] [TRUE, FALSE], "Remote IP"="192.168.8.2", "Vi Path"=w400) -> ()  [unwired: 8 in, 1 out]
                      n196 = call "EnFlo_Error_Handler.vi"("error in (no error)"=errorcluster {"status"=TRUE, "code"=0, "source"="The Aero Server has just attempted to restart the OGI server on the ATE Machine "}, "Error Type"="ATE Machine Pulse Failure", "Dialog Box (T)"=FALSE) -> ()  [unwired: 3 out]
                    }
                    frame "Check Pulse" {
                      n197 = local read "ATE_Machine Status REF"() -> (w418:refnum<k21>)
                      n198 = shared-variable-read(w418) -> (w417:T5)  [unwired: 1 in, 3 out]
                      "ATE_Machine_Status" <- w417
                      n199 = Unbundle By Name(w417) -> ("Pulse"=w406:bool)
                      n200 = while {
                        shift-right: [w441] -> w408
                        shift-left: _ -> [w439]
                        tunnel: w406 -> [w441]
                        shift-left: _ -> [w440]
                        tunnel: [w440] -> w411
                        tunnel: [w439] -> w409
                        shift-left: _ -> [w438]
                        tunnel: [w438] -> w410
                        stop <- TRUE stop-if-true
                      }
                      n201 = Greater?(x=w404, y=3) -> (0:w405:bool)
                      n202 = Select(t=1.0, s=w406, f=0.0) -> (s? t:f=w420:dbl)
                      n203 = case shown="False" w405 {
                        tunnel: [FALSE w431] -> w412
                        tunnel: w411 -> [_ w430]
                        tunnel: w410 -> [_ w429]
                        tunnel: w409 -> [_ w428]
                        tunnel: w408 -> [_ w427]
                        frame False {
                        }
                        frame True {
                          n204 = Build Array(w427, w428, w430, w429) -> (w437:bool[])
                          n205 = Boolean Array To Number(Boolean array=w437) -> (number=w436:u32)
                          n206 = Equal?(x=u32 15, y=w436) -> (x = y?=w432:bool)
                          n207 = Equal?(x=w436, y=u32 0) -> (x = y?=w433:bool)
                          n208 = Or(x=w432, y=w433) -> (x .or. y?=w431:bool)
                        }
                      }
                      n209 = Bundle By Name(cluster=T9 {"Channel Name"="Aero_Tunnel:Server:Pulse", "New Value"=0.0} ("Update Scan Value Cluster"), "New Value"=w420) -> (w422:T9)
                      n210 = Build Array(w422) -> (w421:T9[])
                      n211 = call "Update_Current_Value_client.vi"("Don't Bother with check?"=TRUE, "Update array in"=w421) -> ()
                      n212 = Select(t="Close Server", s=w412, f="End") -> (s? t:f=w415:string)
                      n213 = Increment(x=w404) -> (x+1=w407:i32)
                    }
                    frame "Close Server" {
                      n214 = local read "Paths"() -> (w449:path[])
                      n215 = Index Array(array=w449) -> (element #1=w447:path, element #2=w446:path)  [unwired: 2 in]
                      n216 = call "Close_Remote_Vi.vi"("Also close host?"=FALSE, "Wait after host (ms)"=u32 2000, "Remote IP"="192.168.8.2", "Host Path"=w447, "VI Path"=w446) -> ()  [unwired: 6 in, 1 out]
                    }
                    frame "End" {
                    }
                  }
                }
              }
            }
          }
        }
        n217 = Or(x="Stop Button", y=w43) -> (x .or. y?=w41:bool)
        n218 = case shown="True" w45 {
          tunnel: w47 -> [w65 w91]
          tunnel: w59 -> [w68 w86]
          tunnel: w58 -> [_ w85]
          tunnel: [w66 i64 0 ("Period")] -> w44
          tunnel: w51 -> [w67 w77]
          tunnel: [w63 i64 1 ("Period")] -> w49
          tunnel: w48 -> [w64 w74]
          tunnel: [w68 i64 0 ("Global Start Time")] -> w46
          frame False {
            n219 = case shown="True" w65 {
              tunnel: w67 -> [w69 w71]
              tunnel: [w69 w70] -> w66
              frame False {
              }
              frame True {
                n220 = Increment(x=w71) -> (x+1=w70:i64)
              }
            }
            n221 = Increment(x=w64) -> (x+1=w63:i64)
          }
          frame True {
            n222 = Subtract(x=w86, y=w85) -> (x-y=w84:i64)
            n223 = To Double Precision Float(number=w77) -> (double precision float=w89:dbl)
            n224 = To Double Precision Float(number=w74) -> (double precision float=w79:dbl)
            n225 = To Double Precision Float(number=w84) -> (double precision float=w83:dbl)
            n226 = Divide(x=w89, y=w79) -> (x/y=w88:dbl)
            n227 = Multiply(x=w83, y=1e-09) -> (x*y=w81:dbl)
            n228 = Multiply(x=w88, y=100.0) -> (x*y=w75:dbl)
            n229 = Reciprocal(x=w81) -> (1/x=w80:dbl)
            n230 = local read "OGI Client Loop Status"() -> (w72:T5)
            n231 = Bundle By Name(cluster=w72, "Loop Status"=w91, "Loop Frequency"=w80, "Poor Loops"=w75) -> (→"OGI Client Loop Status":T5)
          }
        }
        n232 = node-c288() -> ()  [unwired: 1 in, 1 out]
      }
      n233 = node-c288(w36) -> ()  [unwired: 1 out]
    }
    frame #3 {
      n234 = local read "ATE_Machine Status REF"() -> (w475:refnum<k21>)
      n235 = local read "Road Control REF"() -> (w470:refnum<k21>)
      n236 = local read "Balance Data REF"() -> (w474:refnum<k21>)
      n237 = local read "Fan Control REF"() -> (w473:refnum<k21>)
      n238 = local read "Road Data REF"() -> (w472:refnum<k21>)
      n239 = local read "Fan Data REF"() -> (w471:refnum<k21>)
      n240 = Close Variable Connection(11:w475) -> ()  [unwired: 1 in, 1 out]
      n241 = Close Variable Connection(11:w474) -> ()  [unwired: 1 in, 1 out]
      n242 = Close Variable Connection(11:w473) -> ()  [unwired: 1 in, 1 out]
      n243 = Close Variable Connection(11:w470) -> ()  [unwired: 1 in, 1 out]
      n244 = Close Variable Connection(11:w471) -> ()  [unwired: 1 in, 1 out]
      n245 = Close Variable Connection(11:w472) -> ()  [unwired: 1 in, 1 out]
      n246 = local read "Paths"() -> (w469:path[])
      n247 = Index Array(array=w469) -> (element #1=w467:path, element #2=w466:path)  [unwired: 2 in]
      n248 = call "Close_Remote_Vi.vi"("Also close host?"=TRUE, "Wait after host (ms)"=u32 2000, "Remote IP"="192.168.8.2", "Host Path"=w467, "VI Path"=w466) -> ()  [unwired: 6 in, 1 out]
    }
  }
